vi "Set Intermediate Buffer.vi"(10 "Intermediate Buffer":refnum<class "DBL Pointer.lvclass">, 11 "Transfer in":refnum<class "Transfer.lvclass">) -> (3 "Transfer out":refnum<class "Transfer.lvclass">)   [LabVIEW 2017, in "DSF Core.lvlib" / "Transfer.lvclass"]
uses:
  Transfer.lvclass
  Pointer/DBL Pointer.lvclass
  Transfer.lvclass/Transfer.ctl
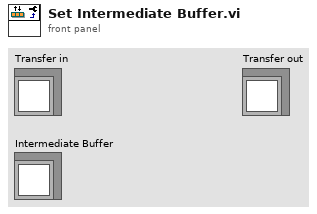
[diagram p1: front panel]
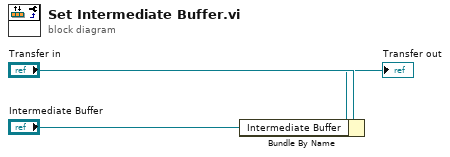
[diagram p0: block diagram]
diagram:
  n1 = Bundle By Name(cluster="Transfer in", "Intermediate Buffer"="Intermediate Buffer") -> (→"Transfer out":refnum<class "Transfer.lvclass">)
